vi "Parse Byte.vi"(6 "Terminal Options":T2={"Implied CR with LF"=TRUE, "Local Echo"=FALSE, "Tab Width"=8, "Color Scheme"={"Black"=2302755, "Red"=16711695, "Green"=9232651, "Yellow"=16759040, "Blue"=36344, "Magenta"=7160742, "Cyan"=55531, "White"=15132390, "Bright Black"=4473924, "Bright Red"=16721728, "Bright Green"=11264347, "Bright Yellow"=16765506, "Bright Blue"=37631, "Bright Magenta"=10117099, "Bright Cyan"=6815728, "Bright White"=16777215}, "Default FG"=37, "Default BG"=90, "History Length"=5000, "Font Face"="", "Font Size"=14, "Rows"=24, "Cols"=80} {"Default BG" items=["Black"=30, "Red"=31, "Green"=32, "Yellow"=33, "Blue"=34, "Magenta"=35, "Cyan"=36, "White"=37, "Gray"=90, "Bright Red"=91, "Bright Green"=92, "Bright Yellow"=93, "Bright Blue"=94, "Bright Magenta"=95, "Bright Cyan"=96, "Bright White"=97]; "Default FG" items=["Black"=30, "Red"=31, "Green"=32, "Yellow"=33, "Blue"=34, "Magenta"=35, "Cyan"=36, "White"=37, "Gray"=90, "Bright Red"=91, "Bright Green"=92, "Bright Yellow"=93, "Bright Blue"=94, "Bright Magenta"=95, "Bright Cyan"=96, "Bright White"=97]}, 7 "Buffers":T1, 10 "Byte":u8, 11 "Parse State In":T5) -> (2 "Bell":bool, 3 "Parse State":T5)   [LabVIEW 2020, in "Terminal.lvlib" / "Terminal.lvclass"]
uses:
  Terminal.lvclass
  Parse State.ctl
  Buffer State.ctl
  Cursor.ctl
  Position.ctl
  Text Attributes.ctl
  Terminal Options.ctl
  Color Scheme.ctl
  Color.ctl
  Buffers.ctl
  TermBuffer/TermBuffer.lvclass
  Terminal.lvclass/Terminal.ctl
  Terminal.lvlib
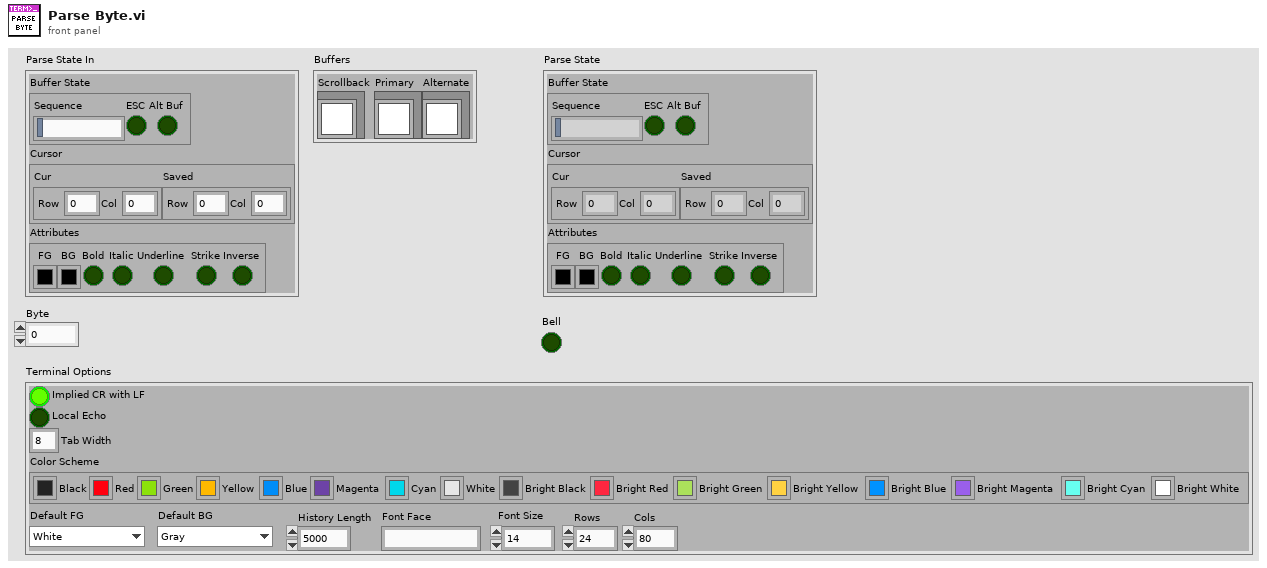
[diagram p1: front panel]
types:
  T1 = typedef "Terminal.lvlib/Terminal.lvclass/Buffers.ctl" = cluster{"Scrollback":refnum<class "TermBuffer.lvclass">, "Primary":refnum<class "TermBuffer.lvclass">, "Alternate":refnum<class "TermBuffer.lvclass">}
  T2 = typedef "Terminal.lvlib/Terminal Options.ctl" = cluster{"Implied CR with LF":bool, "Local Echo":bool, "Tab Width":i32, "Color Scheme":T3, "Default FG":T4, "Default BG":T4, "History Length":i32, "Font Face":string, "Font Size":i16, "Rows":i32, "Cols":i32}
  T3 = typedef "Terminal.lvlib/Color Scheme.ctl" = cluster{"Black":u32, "Red":u32, "Green":u32, "Yellow":u32, "Blue":u32, "Magenta":u32, "Cyan":u32, "White":u32, "Bright Black":u32, "Bright Red":u32, "Bright Green":u32, "Bright Yellow":u32, "Bright Blue":u32, "Bright Magenta":u32, "Bright Cyan":u32, "Bright White":u32}
  T4 = typedef "Terminal.lvlib/Color.ctl" = i8
  T5 = typedef "Terminal.lvlib/Terminal.lvclass/Parse State.ctl" = cluster{"Buffer State":T6, "Cursor":T7, "Attributes":T9}
  T6 = typedef "Terminal.lvlib/Terminal.lvclass/Buffer State.ctl" = cluster{"Sequence":string, "ESC":bool, "Alt Buf":bool}
  T7 = typedef "Terminal.lvlib/Terminal.lvclass/Cursor.ctl" = cluster{"Cur":T8, "Saved":T8}
  T8 = typedef "Terminal.lvlib/Terminal.lvclass/Position.ctl" = cluster{"Row":i32, "Col":i32}
  T9 = typedef "Terminal.lvlib/Text Attributes.ctl" = cluster{"FG":u32, "BG":u32, "Bold":bool, "Italic":bool, "Underline":bool, "Strike":bool, "Inverse":bool}
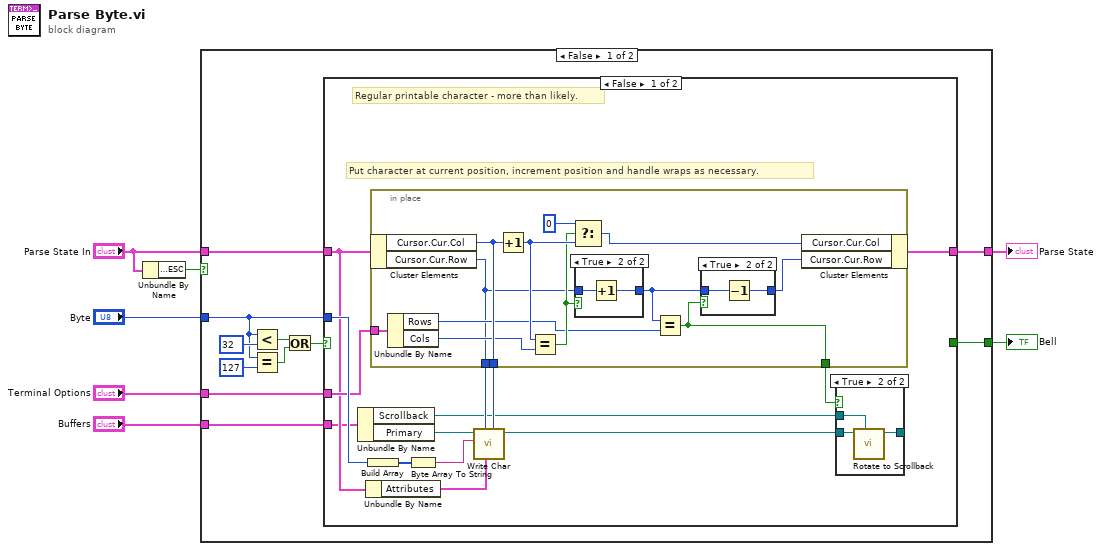
[diagram p0: block diagram]
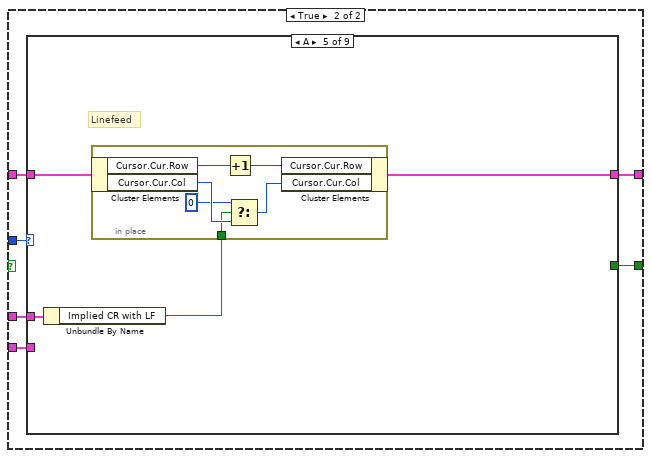
[diagram p5: hidden frame]
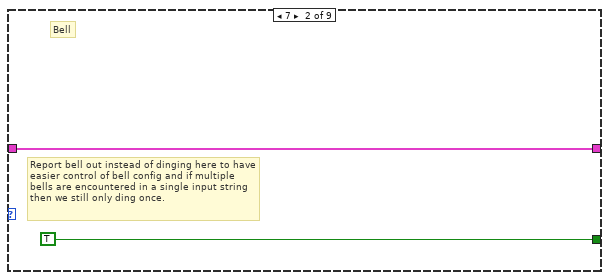
[diagram p7: hidden frame]
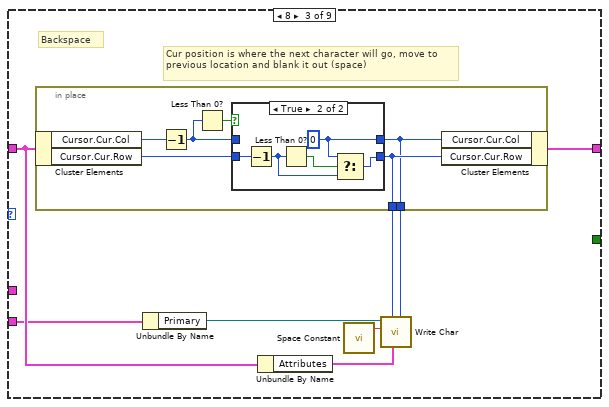
[diagram p8: hidden frame]
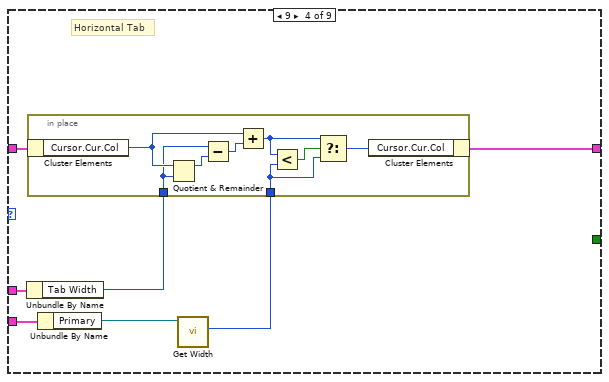
[diagram p10: hidden frame]
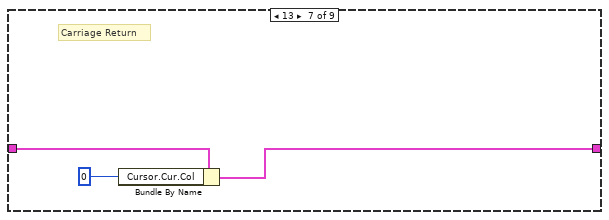
[diagram p12: hidden frame]
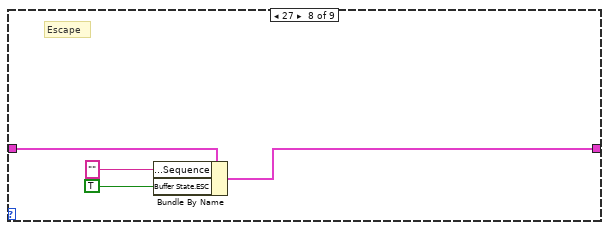
[diagram p13: hidden frame]
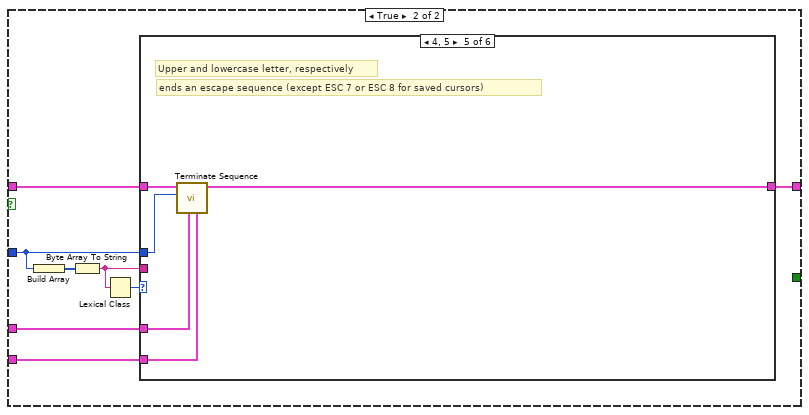
[diagram p15: hidden frame]
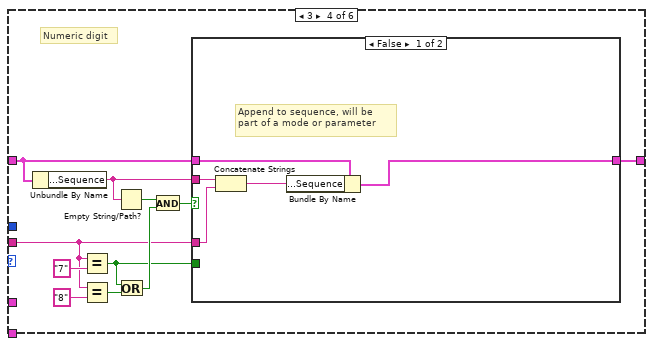
[diagram p19: hidden frame]
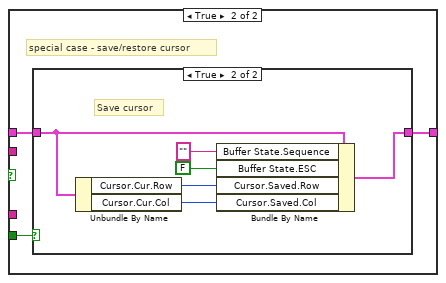
[diagram p20: hidden frame]
diagram:
  n1 = Unbundle By Name("Parse State In") -> ("Buffer State.ESC"=w5:bool)
  n2 = case shown="False" w5 {
    tunnel: "Byte" -> [w13 w121]
    tunnel: [w12 _] -> w6
    tunnel: "Parse State In" -> [w11 w123]
    tunnel: [w10 w122] -> w3
    tunnel: "Terminal Options" -> [w9 w120]
    tunnel: "Buffers" -> [w8 w119]
    frame False {
      n3 = Less?(x=w13, y=u8 32) -> (x < y?=w16:bool)
      n4 = Equal?(x=w13, y=u8 127) -> (x = y?=w14:bool)
      n5 = Or(x=w16, y=w14) -> (x .or. y?=w15:bool)
      n6 = case shown="False" w15 {
        tunnel: w13 -> [w32 w60]
        tunnel: [_ w59] -> w12
        tunnel: w11 -> [w28 w58]
        tunnel: [w24 w57] -> w10
        tunnel: w9 -> [w29 w56]
        tunnel: w8 -> [w23 w55]
        frame False {
          # "Put character at current position, increment position and handle wraps as necessary."
          # "Regular printable character - more than likely."
          n7 = Unbundle By Name(w23) -> ("Scrollback"=w22:refnum<class "TermBuffer.lvclass">, "Primary"=w20:refnum<class "TermBuffer.lvclass">)
          n8 = Unbundle By Name(w28) -> ("Attributes"=w27:T9)
          n9 = Build Array(w32) -> (w31:u8[])
          n10 = in-place {
            in-place-border: w29 -> [w48]
            in-place-border: [w40] -> w26
            in-place-border: [w47] -> w25
            in-place-border: [w38] -> w21
            n11 = in-place-cluster #1(w28) -> ("Cursor.Cur.Col"=w47:i32, "Cursor.Cur.Row"=w40:i32)
            n12 = Unbundle By Name(w48) -> ("Rows"=w41:i32, "Cols"=w46:i32)
            n13 = Increment(x=w47) -> (x+1=w45:i32)
            n14 = Equal?(x=w45, y=w46) -> (x = y?=w42:bool)
            n15 = Select(t=0, s=w42, f=w45) -> (s? t:f=w43:i32)
            n16 = case shown="True" w42 {
              tunnel: w40 -> [w52 w54]
              tunnel: [w52 w53] -> w39
              frame False {
              }
              frame True {
                n17 = Increment(x=w54) -> (x+1=w53:i32)
              }
            }
            n18 = Equal?(x=w39, y=w41) -> (x = y?=w38:bool)
            n19 = case shown="True" w38 {
              tunnel: w39 -> [w49 w51]
              tunnel: [w49 w50] -> w37
              frame False {
              }
              frame True {
                n20 = Decrement(x=w51) -> (x-1=w50:i32)
              }
            }
            n21 = in-place-cluster #1("Cursor.Cur.Col"=w43, "Cursor.Cur.Row"=w37) -> (w24:T5)
          }
          n22 = Byte Array To String(unsigned byte array=w31) -> (string=w30:string)
          n23 = call "Write Char.vi"("Col"=w25, "Attributes"=w27, "Row"=w26, "Char"=w30, "TermBuffer in"=w20) -> ("TermBuffer out"=w19:refnum<class "TermBuffer.lvclass">)  [unwired: 5 in, 1 out]
          n24 = case shown="True" w21 {
            tunnel: w22 -> [_ w36]
            tunnel: w19 -> [w33 w35]
            tunnel: [w33 w34] -> _
            frame False {
            }
            frame True {
              n25 = call "Rotate to Scrollback.vi"("Scrollback"=w36, "TermBuffer in"=w35) -> ("TermBuffer out"=w34:refnum<class "TermBuffer.lvclass">)  [unwired: 8 in, 1 out]
            }
          }
        }
        frame True {
          n26 = case shown="A" w60 {
            tunnel: [_ TRUE _ _ _ _ _ _ _] -> w59
            tunnel: w58 -> [w61 w62 w71 w90 w102 w110 w113 w117 w118]
            tunnel: [w61 w62 w68 w89 w100 w110 w111 w114 w118] -> w57
            tunnel: w56 -> [_ _ _ w88 w103 _ _ _ _]
            tunnel: w55 -> [_ _ w65 w86 _ _ _ _ _]
            frame Default {
              # "Unknown / Unhandled"
            }
            frame 7 {
              # "Bell"
              # "Report bell out instead of dinging here to have easier control of bell config and if multiple bells are encountered in a single input string then we still only ding once."
            }
            frame 8 {
              # "Cur position is where the next character will go, move to previous location and blank it out (space)"
              # "Backspace"
              n27 = in-place {
                in-place-border: [w73] -> w67
                in-place-border: [w72] -> w66
                n28 = in-place-cluster #2(w71) -> ("Cursor.Cur.Col"=w77:i32, "Cursor.Cur.Row"=w74:i32)
                n29 = Decrement(x=w77) -> (x-1=w75:i32)
                n30 = Less Than 0?(x=w75) -> (x < 0?=w76:bool)
                n31 = case shown="True" w76 {
                  tunnel: w75 -> [w79 _]
                  tunnel: w74 -> [w78 w84]
                  tunnel: [w79 w81] -> w72
                  tunnel: [w78 w80] -> w73
                  frame False {
                  }
                  frame True {
                    w81 = 0 ("f")
                    n32 = Decrement(x=w84) -> (x-1=w83:i32)
                    n33 = Less Than 0?(x=w83) -> (x < 0?=w82:bool)
                    n34 = Select(t=w81, s=w82, f=w83) -> (s? t:f=w80:i32)
                  }
                }
                n35 = in-place-cluster #2("Cursor.Cur.Col"=w72, "Cursor.Cur.Row"=w73) -> (w68:T5)
              }
              n36 = Unbundle By Name(w65) -> ("Primary"=w64:refnum<class "TermBuffer.lvclass">)
              n37 = Unbundle By Name(w71) -> ("Attributes"=w70:T9)
              n38 = call <vilib>:"Space Constant.vi"() -> ("String"=w69:string)
              n39 = call "Write Char.vi"("Col"=w66, "Attributes"=w70, "Row"=w67, "Char"=w69, "TermBuffer in"=w64) -> ()  [unwired: 5 in, 2 out]
            }
            frame 9 {
              # "Horizontal Tab"
              n40 = Unbundle By Name(w88) -> ("Tab Width"=w87:i32)
              n41 = Unbundle By Name(w86) -> ("Primary"=w85:refnum<class "TermBuffer.lvclass">)
              n42 = call "Get Width.vi"("TermBuffer in"=w85) -> ("Width"=w91:i32)  [unwired: 8 in, 2 out]
              n43 = in-place {
                in-place-border: w91 -> [w95]
                in-place-border: w87 -> [w92]
                n44 = in-place-cluster #3(w90) -> ("Cursor.Cur.Col"=w93:i32)
                n45 = Quotient & Remainder(x=w93, y=w92) -> (x-y*floor(x/y)=w99:i32)  [unwired: 1 out]
                n46 = Subtract(x=w92, y=w99) -> (x-y=w98:i32)
                n47 = Add(x=w93, y=w98) -> (x+y=w97:i32)
                n48 = Less?(x=w97, y=w95) -> (x < y?=w96:bool)
                n49 = Select(t=w97, s=w96, f=w95) -> (s? t:f=w94:i32)
                n50 = in-place-cluster #3("Cursor.Cur.Col"=w94) -> (w89:T5)
              }
            }
            frame 10 {
              # "Linefeed"
              n51 = Unbundle By Name(w103) -> ("Implied CR with LF"=w101:bool)
              n52 = in-place {
                in-place-border: w101 -> [w106]
                n53 = in-place-cluster #4(w102) -> ("Cursor.Cur.Row"=w109:i32, "Cursor.Cur.Col"=w108:i32)
                n54 = Increment(x=w109) -> (x+1=w104:i32)
                n55 = Select(t=0 ("f"), s=w106, f=w108) -> (s? t:f=w105:i32)
                n56 = in-place-cluster #4("Cursor.Cur.Row"=w104, "Cursor.Cur.Col"=w105) -> (w100:T5)
              }
            }
            frame 12 {
              # "Do nothing for now"
              # "Formfeed"
            }
            frame 13 {
              # "Carriage Return"
              n57 = Bundle By Name(cluster=w113, "Cursor.Cur.Col"=0 ("Cur Col")) -> (w111:T5)
            }
            frame 27 {
              # "Escape"
              n58 = Bundle By Name(cluster=w117, "Buffer State.Sequence"="" ("Sequence"), "Buffer State.ESC"=TRUE ("ESC")) -> (w114:T5)
            }
            frame 127 {
              # "Delete"
            }
          }
        }
      }
    }
    frame True {
      n59 = Build Array(w121) -> (w126:u8[])
      n60 = Byte Array To String(unsigned byte array=w126) -> (string=w124:string)
      n61 = Lexical Class(1:w124) -> (0:w125:i16)
      n62 = case shown="4, 5" w125 {
        tunnel: w124 -> [_ _ _ w130 _ w167]
        tunnel: w123 -> [w127 w128 w129 w133 w165 w168]
        tunnel: [w127 w128 w129 w131 w164 w166] -> w122
        tunnel: w121 -> [_ _ _ _ w163 _]
        tunnel: w120 -> [_ _ _ _ w162 _]
        tunnel: w119 -> [_ _ _ _ w161 _]
        frame Default {
        }
        frame 0, 1 {
          # "#ERROR?\nSome terminals immediately stop processing escape sequences, some ignore unexpected characters, and others complete the sequence but ignore the sequence with bad chars... which should we do?"
          # "Extended ascii & Non-displayable, respectively"
        }
        frame 2 {
          # "Whitespace can be ignored in escape sequences and is only present for readability."
          # "Whitespace"
        }
        frame 3 {
          # "Numeric digit"
          n63 = Unbundle By Name(w133) -> ("Buffer State.Sequence"=w134:string)
          n64 = Equal?(x=w130, y="7") -> (x = y?=w132:bool)
          n65 = Equal?(x=w130, y="8") -> (x = y?=w138:bool)
          n66 = Empty String/Path?(string/path=w134) -> (empty?=w137:bool)
          n67 = Or(x=w132, y=w138) -> (x .or. y?=w136:bool)
          n68 = And(x=w137, y=w136) -> (x .and. y?=w135:bool)
          n69 = case shown="False" w135 {
            tunnel: w134 -> [w144 _]
            tunnel: w133 -> [w143 w147]
            tunnel: w132 -> [_ w148]
            tunnel: [w141 w146] -> w131
            tunnel: w130 -> [w145 _]
            frame False {
              # "Append to sequence, will be part of a mode or parameter"
              n70 = Concatenate Strings(w144, w145) -> (w142:string)
              n71 = Bundle By Name(cluster=w143, "Buffer State.Sequence"=w142) -> (w141:T5)
            }
            frame True {
              # "special case - save/restore cursor"
              n72 = case shown="True" w148 {
                tunnel: w147 -> [w151 w157]
                tunnel: [w152 w158] -> w146
                frame False {
                  # "Restore saved cursor"
                  n73 = Unbundle By Name(w151) -> ("Cursor.Saved.Row"=w150:i32, "Cursor.Saved.Col"=w149:i32)
                  n74 = Bundle By Name(cluster=w151, "Buffer State.Sequence"="" ("Sequence"), "Buffer State.ESC"=FALSE ("ESC"), "Cursor.Cur.Row"=w150, "Cursor.Cur.Col"=w149) -> (w152:T5)
                }
                frame True {
                  # "Save cursor"
                  n75 = Unbundle By Name(w157) -> ("Cursor.Cur.Row"=w156:i32, "Cursor.Cur.Col"=w155:i32)
                  n76 = Bundle By Name(cluster=w157, "Buffer State.Sequence"="" ("Sequence"), "Buffer State.ESC"=FALSE ("ESC"), "Cursor.Saved.Row"=w156, "Cursor.Saved.Col"=w155) -> (w158:T5)
                }
              }
            }
          }
        }
        frame 4, 5 {
          # "ends an escape sequence (except ESC 7 or ESC 8 for saved cursors)"
          # "Upper and lowercase letter, respectively"
          n77 = call "Terminate Sequence.vi"("Buffers"=w161, "Terminal Options"=w162, "Terminator"=w163, "Parse State In"=w165) -> ("Parse State"=w164:T5)  [unwired: 7 in]
        }
        frame 6 {
          # "Contains some characters such as ; which are used to characterize sequences and separate arguments."
          # "Printable non-alphanumeric"
          n78 = in-place {
            in-place-border: w167 -> [w169]
            n79 = in-place-cluster #5(w168) -> ("Buffer State.Sequence"=w171:string)
            n80 = Concatenate Strings(w171, w169) -> (w170:string)
            n81 = in-place-cluster #5("Buffer State.Sequence"=w170) -> (w166:T5)
          }
        }
      }
    }
  }
  "Parse State" <- w3
  "Bell" <- w6
